vi "Error Test Start Bit Value.vi"(6 "error text in":string, 7 "direction":T1, 8 "error in":errorcluster, 9 "start bit":i32) -> (0 "error out":errorcluster)   [LabVIEW 2023]
uses:
  Direction.ctl
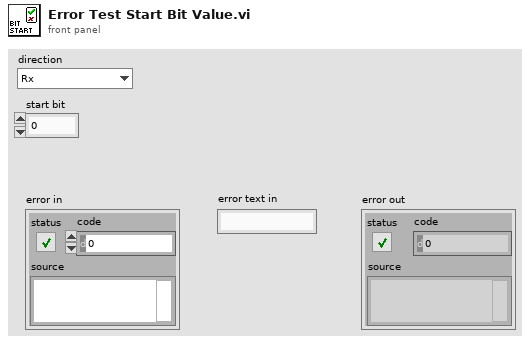
[diagram p1: front panel]
types:
  T1 = typedef "Direction.ctl" = enum16{"Rx", "Tx"}
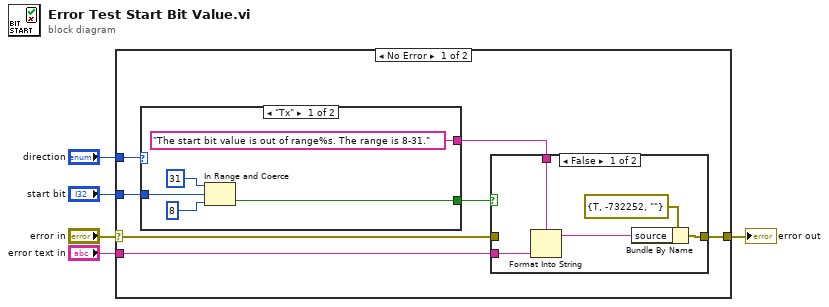
[diagram p0: block diagram]
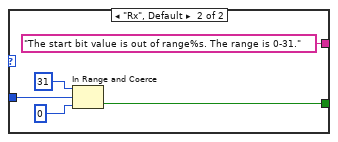
[diagram p2: hidden frame]
diagram:
  n1 = case shown="No Error" "error in" {
    selector: "error in" -> [w11 w29]
    tunnel: [w10 w29] -> w4
    tunnel: "start bit" -> [w12 _]
    tunnel: "error text in" -> [w9 _]
    tunnel: "direction" -> [w7 _]
    frame No Error {
      n2 = case shown="\"Tx\"" w7 {
        tunnel: w12 -> [w17 w22]
        tunnel: [w14 w19] -> w8
        tunnel: ["The start bit value is out of range%s. The range is 8-31." ("source") "The start bit value is out of range%s. The range is 0-31." ("source")] -> w6
        frame "Tx" {
          n3 = In Range and Coerce(upper limit=31 ("lower limit"), x=w17, lower limit=8) -> (In Range?=w14:bool)  [unwired: 1 out]
        }
        frame "Rx", Default {
          n4 = In Range and Coerce(upper limit=31 ("lower limit"), x=w22, lower limit=0) -> (In Range?=w19:bool)  [unwired: 1 out]
        }
      }
      n5 = case shown="False" w8 {
        tunnel: w11 -> [_ w28]
        tunnel: [w27 w28] -> w10
        tunnel: w9 -> [w25 _]
        tunnel: w6 -> [w23 _]
        frame False {
          n6 = Format Into String(format string=w23, w25) -> (resulting string=w26:string)  [unwired: 2 in, 1 out]
          n7 = Bundle By Name(cluster=errorcluster {"status"=TRUE, "code"=-732252, "source"=""} ("error constant"), "source"=w26) -> (w27:errorcluster)
        }
        frame True {
        }
      }
    }
    frame Error {
    }
  }
  "error out" <- w4
